vi "Draw Breadcrumb.vi"(8 "error in (no error)":errorcluster, 11 "BreadcrumbNavigation in":refnum<class "BreadcrumbNavigator.lvclass">) -> (0 "error out":errorcluster, 3 "BreadcrumbNavigation out":refnum<class "BreadcrumbNavigator.lvclass">)   [LabVIEW 2015, in "BreadcrumbNavigator.lvclass"]
uses:
  BreadcrumbNavigator.lvclass
  BreadcrumbNavigator.lvclass/BreadcrumbNavigator.ctl
  Read Delimeter.vi
  Read Strings[].vi
  Write CurrentLeftMostItem.vi
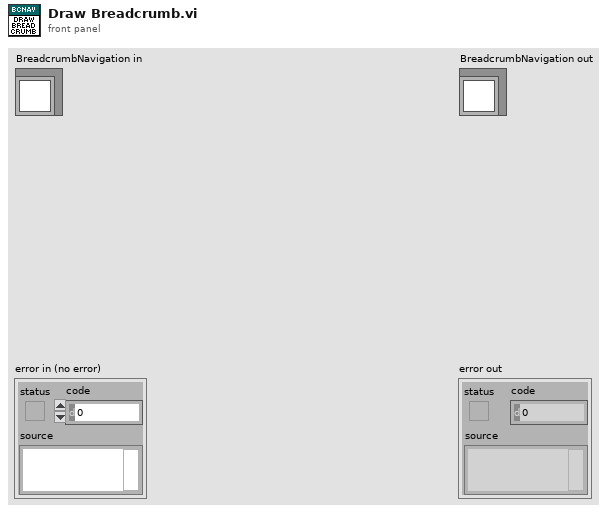
[diagram p1: front panel]
types:
  T1 = enum16{"User-specified Font", "Application Font", "System Font", "Dialog Font"}
  T2 = typedef "LVFontTypeDef.ctl" = cluster{"Font Name":string, "Size":u16, "Bold":bool, "Italic":bool, "Underline":bool, "Strikeout":bool, "Color":u32}
  T3 = cluster{"Font Name:":string, "Size":i16, "Strikeout?":bool, "Italic?":bool, "Underline?":bool, "Outline?":bool, "Shadow?":bool, "Bold?":bool}
  T4 = cluster{"left":i16, "top":i16, "right":i16, "bottom":i16}
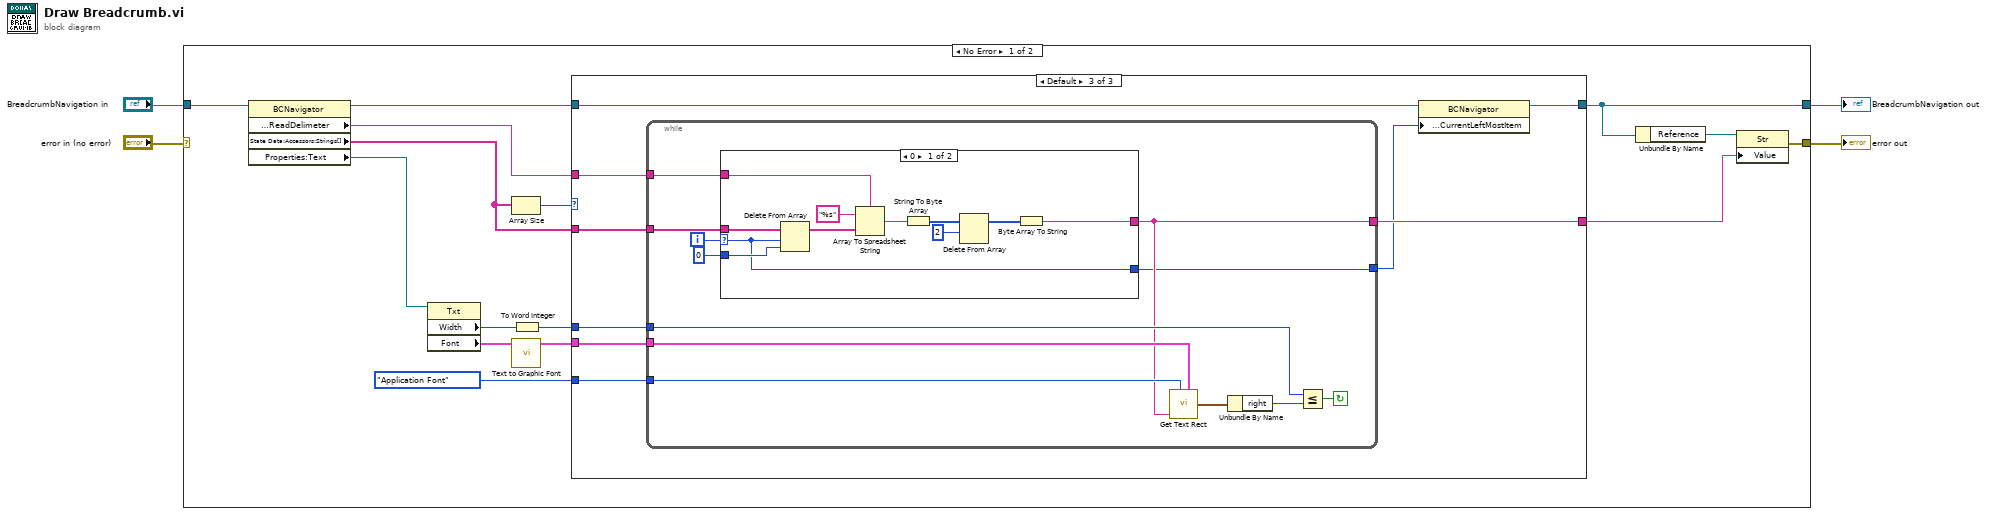
[diagram p0: block diagram]
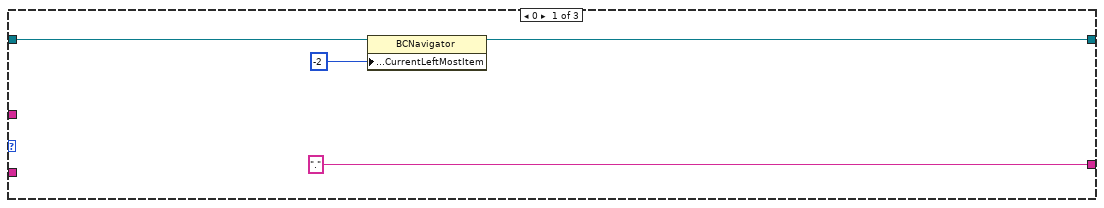
[diagram p2: hidden frame]
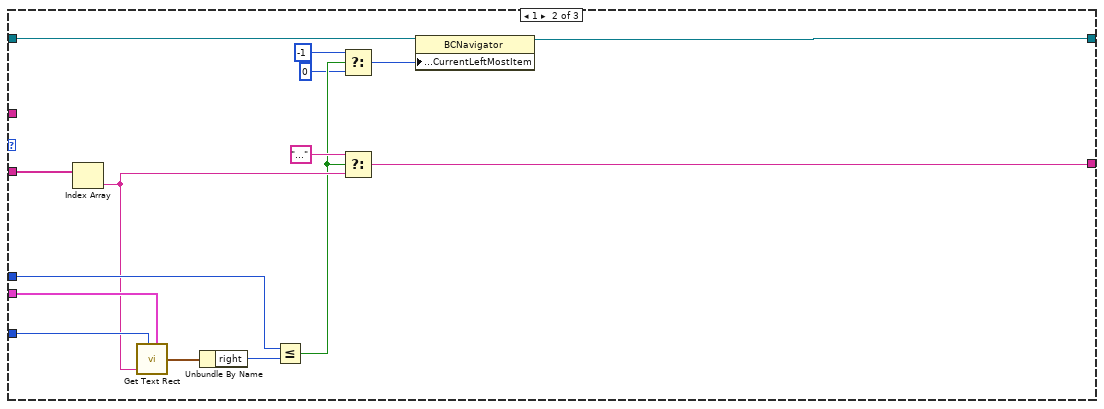
[diagram p3: hidden frame]
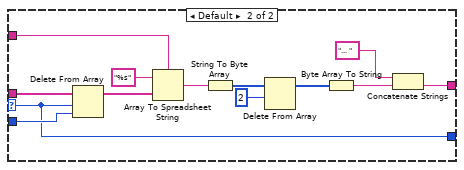
[diagram p4: hidden frame]
diagram:
  n1 = case shown="No Error" "error in (no error)" {
    selector: "error in (no error)" -> [_ w85]
    tunnel: [w6 w85] -> w3
    tunnel: [w9 w84] -> w1
    tunnel: "BreadcrumbNavigation in" -> [w19 w84]
    frame No Error {
      n2 = property class="BCNavigator"(reference=w19) -> (reference out=w11:refnum<class "BreadcrumbNavigator.lvclass">, "State Data:Accessors:ReadDelimeter"=w5:string, "State Data:Accessors:Strings[]"=w10:string[], "Properties:Text"=w18:refnum<vi>)  [unwired: 1 in, 1 out]
      n3 = property class="Txt"(reference=w18) -> ("Width"=w17:u32, "Font"=w15:T2)  [unwired: 1 in, 2 out]
      n4 = Array Size(array=w10) -> (size(s)=w12:i32)
      n5 = call "Text to Graphic Font.vi"("Text Font"=w15) -> ("Graphic Font"=w14:T3)  [unwired: 10 in]
      n6 = To Word Integer(number=w17) -> (16bit integer=w13:i16)
      n7 = case shown="Default" w12 {
        tunnel: w10 -> [_ w33 w43]
        tunnel: T1."Application Font" ("desired font(Application)") -> [_ w38 w47]
        tunnel: w14 -> [_ w37 w46]
        tunnel: w13 -> [_ w36 w45]
        tunnel: ["." w30 w41] -> w7
        tunnel: w11 -> [w22 w29 w44]
        tunnel: [w20 w24 w42] -> w9
        tunnel: w5 -> [_ _ w39]
        frame 0 {
          n8 = property class="BCNavigator"(reference=w22, "State Data:Accessors:CurrentLeftMostItem"=-2 ("CurrentLeftMostItem")) -> (reference out=w20:refnum<class "BreadcrumbNavigator.lvclass">)  [unwired: 1 in, 1 out]
        }
        frame 1 {
          n9 = Index Array(array=w33) -> (element=w32:string)  [unwired: 1 in]
          n10 = call <vilib>:"Get Text Rect.vi"("desired font(Application)"=w38, "text"=w32, "[user-specified font]"=w37) -> ("rect"=w35:T4)  [unwired: 6 in]
          n11 = Unbundle By Name(w35) -> ("right"=w34:i16)
          n12 = Less Or Equal?(x=w36, y=w34) -> (x <= y?=w28:bool)
          n13 = Select(t=-1, s=w28, f=0) -> (s? t:f=w25:i32)
          n14 = Select(t="...", s=w28, f=w32) -> (s? t:f=w30:string)
          n15 = property class="BCNavigator"(reference=w29, "State Data:Accessors:CurrentLeftMostItem"=w25) -> (reference out=w24:refnum<class "BreadcrumbNavigator.lvclass">)  [unwired: 1 in, 1 out]
        }
        frame Default {
          n16 = while {
            tunnel: w45 -> [w55]
            tunnel: w47 -> [w59]
            tunnel: w46 -> [w58]
            tunnel: w43 -> [w53]
            tunnel: [w52] -> w41
            tunnel: [w49] -> w40
            tunnel: w39 -> [w48]
            i -> [w51]
            stop <- w54 continue-if-true
            n17 = case shown="0" w51 {
              selector: w51 -> [w61 w72]
              tunnel: w53 -> [w70 w83]
              tunnel: [w64 w74] -> w52
              tunnel: 0 ("index") -> [w62 w75]
              tunnel: [w61 w72] -> w49
              tunnel: w48 -> [w60 w71]
              frame 0 {
                n18 = Delete From Array(array=w70, length=w61, index=w62) -> (array with subset deleted=w63:string[])  [unwired: 1 out]
                n19 = Array To Spreadsheet String(delimiter (Tab)=w60, array=w63, 3:"%s" ("format string")) -> (spreadsheet string=w68:string)
                n20 = String To Byte Array(string=w68) -> (unsigned byte array=w67:u8[])
                n21 = Delete From Array(array=w67, length=2) -> (array with subset deleted=w65:u8[])  [unwired: 1 in, 1 out]
                n22 = Byte Array To String(unsigned byte array=w65) -> (string=w64:string)
              }
              frame Default {
                n23 = Delete From Array(array=w83, length=w72, index=w75) -> (array with subset deleted=w76:string[])  [unwired: 1 out]
                n24 = Array To Spreadsheet String(delimiter (Tab)=w71, array=w76, 3:"%s" ("format string")) -> (spreadsheet string=w81:string)
                n25 = String To Byte Array(string=w81) -> (unsigned byte array=w80:u8[])
                n26 = Delete From Array(array=w80, length=2) -> (array with subset deleted=w78:u8[])  [unwired: 1 in, 1 out]
                n27 = Byte Array To String(unsigned byte array=w78) -> (string=w77:string)
                n28 = Concatenate Strings("... " ("string"), w77) -> (w74:string)
              }
            }
            n29 = call <vilib>:"Get Text Rect.vi"("desired font(Application)"=w59, "text"=w52, "[user-specified font]"=w58) -> ("rect"=w57:T4)  [unwired: 6 in]
            n30 = Unbundle By Name(w57) -> ("right"=w56:i16)
            n31 = Less Or Equal?(x=w55, y=w56) -> (x <= y?=w54:bool)
          }
          n32 = property class="BCNavigator"(reference=w44, "State Data:Accessors:CurrentLeftMostItem"=w40) -> (reference out=w42:refnum<class "BreadcrumbNavigator.lvclass">)  [unwired: 1 in, 1 out]
        }
      }
      n33 = Unbundle By Name(w9) -> ("Reference"=w8:refnum<vi>)
      n34 = property class="Str"(reference=w8, "Value"=w7) -> (error out=w6:errorcluster)  [unwired: 1 in, 1 out]
    }
    frame Error {
    }
  }
  "error out" <- w3
  "BreadcrumbNavigation out" <- w1
